vi "KillWaves.vi"(8 "error in (no error)":errorcluster, 10 "wavename":string, 11 "ITX Commands in":refnum<class "ITX Commands.lvclass">) -> (0 "error out":errorcluster, 3 "ITX Commands out":refnum<class "ITX Commands.lvclass">)   [LabVIEW 2019, in "ITX Commands.lvclass"]
uses:
  ITX Commands.lvclass
panel:
  out "Command String":string
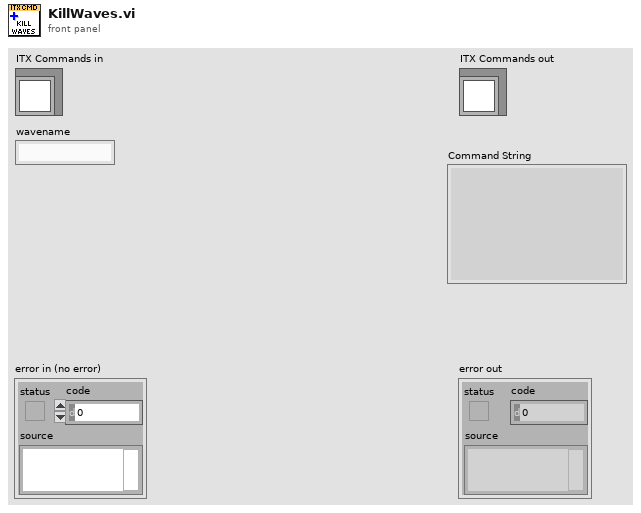
[diagram p1: front panel]
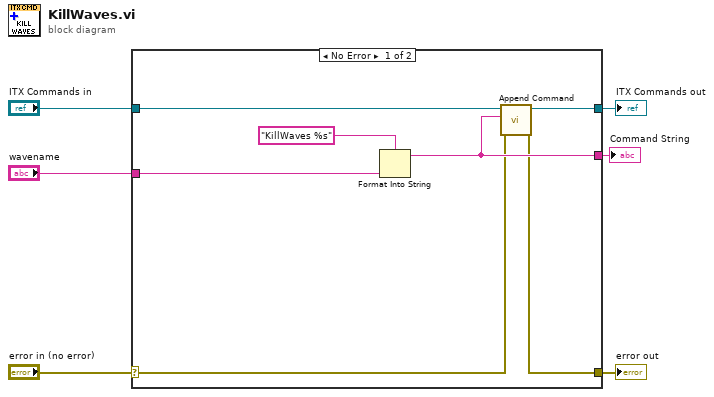
[diagram p0: block diagram]
diagram:
  n1 = case shown="No Error" "error in (no error)" {
    selector: "error in (no error)" -> [w8 w15]
    tunnel: [w7 w15] -> w5
    tunnel: [w10 w14] -> w3
    tunnel: "ITX Commands in" -> [w9 w14]
    tunnel: "wavename" -> [w12 _]
    tunnel: [w11 _] -> w1
    frame No Error {
      n2 = Format Into String(format string="KillWaves %s" ("input string 1"), w12) -> (resulting string=w11:string)  [unwired: 2 in, 1 out]
      n3 = call "Append Command.vi"("error in (no error)"=w8, "New Command"=w11, "ITX Commands in"=w9) -> ("error out"=w7:errorcluster, "ITX Commands out"=w10:refnum<class "ITX Commands.lvclass">)  [unwired: 7 in]
    }
    frame Error {
    }
  }
  "error out" <- w5
  "ITX Commands out" <- w3
  "Command String" <- w1
